vi "process.vi"(8 "error in (no error)":errorcluster, 11 "VI in":refnum<class "VI.lvclass">) -> (0 "error out":errorcluster, 3 "VI out":refnum<class "VI.lvclass">)   [LabVIEW 2016, in "VI.lvclass"]
uses:
  VI.lvclass
  C:/LSST_TS/SystemSW/ct_tools/ProjectItem/ProjectItem.lvclass
  ProjectItem/ProjectItem.lvclass/ProjectItem.ctl
  ProjectItem/ProjectItem.lvclass
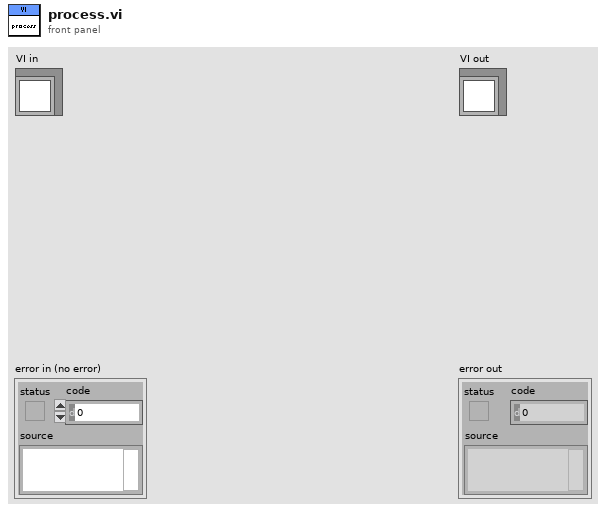
[diagram p1: front panel]
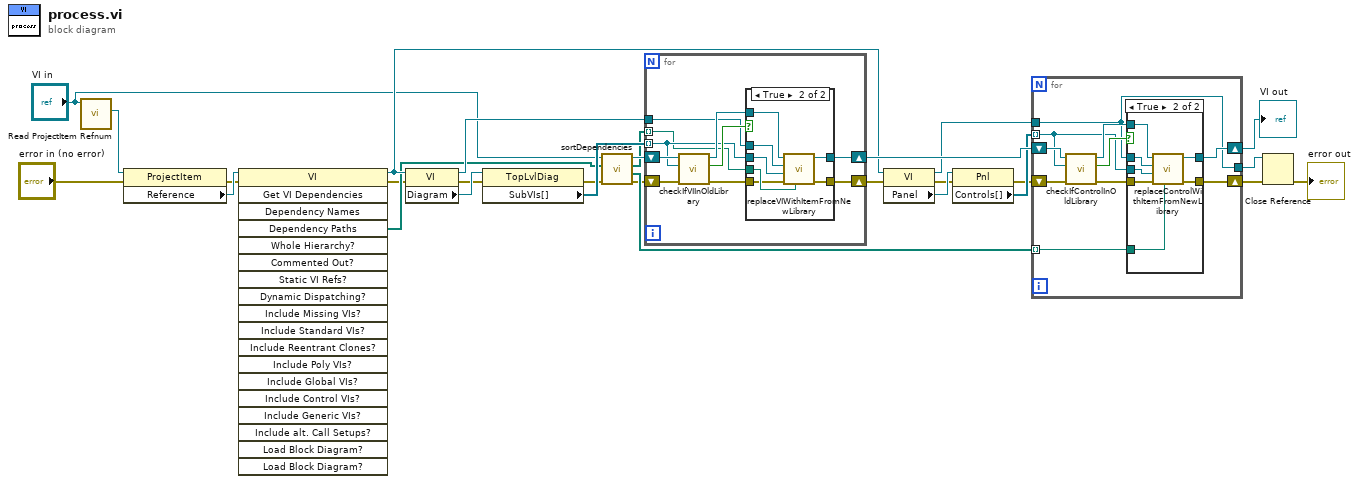
[diagram p0: block diagram]
diagram:
  n1 = call "Read ProjectItem Refnum.vi"("ProjectItem in"="VI in") -> ("ProjectItem Refnum"=w26:refnum<vi>)  [unwired: 9 in, 1 out]
  n2 = property class="ProjectItem"(reference=w26, error in="error in (no error)") -> (error out=w11:errorcluster, "Reference"=w25:refnum<vi>)  [unwired: 1 out]
  n3 = invoke class="VI" method="Get VI Dependencies"(reference=w25, error in=w11) -> (reference out=w20:refnum<vi>, error out=w10:errorcluster, "Dependency Paths"=w15:path[])  [unwired: 17 in, 16 out]
  n4 = property class="VI"(reference=w20, error in=w10) -> (reference out=w24:refnum<vi>, error out=w9:errorcluster, "Diagram"=w28:refnum<vi>)
  n5 = property class="TopLvlDiag"(reference=w28, error in=w9) -> (error out=w8:errorcluster, "SubVIs[]"=w27:refnum<vi>[])  [unwired: 1 out]
  n6 = call "sortDependencies.vi"("error in (no error)"=w8, "Dependency Paths"=w15, "VI in"="VI in") -> ("error out"=w7:errorcluster, "ControlDependencyPaths"=w13:path[], "VIDependencyPaths"=w14:path[], "VI out"=w16:refnum<class "VI.lvclass">)  [unwired: 5 in]
  n7 = for {
    shift-right: [w36] -> w22
    shift-left: w16 -> [w38]
    tunnel: w27 -> [w33] mode=indexing
    tunnel: w24 -> [w34]
    tunnel: w14 -> [w32] mode=indexing
    shift-right: [w29] -> w6
    shift-left: w7 -> [w31]
    n8 = call "checkIfVIInOldLibrary.vi"("error in (no error)"=w31, "element"=w33, "VI in"=w38) -> ("error out"=w30:errorcluster, "isMemberOfOldLibrary"=w35:bool, "VI out"=w37:refnum<class "VI.lvclass">)  [unwired: 5 in, 1 out]
    n9 = case shown="True" w35 {
      tunnel: w37 -> [w40 w47]
      tunnel: [w40 w46] -> w36
      tunnel: w34 -> [_ w45]
      tunnel: w33 -> [_ w44]
      tunnel: w32 -> [_ w43]
      tunnel: w30 -> [w39 w42]
      tunnel: [w39 w41] -> w29
      frame False {
      }
      frame True {
        n10 = call "replaceVIWithItemFromNewLibrary.vi"("SubVI Path"=w43, "error in (no error)"=w42, "SubVI Refnum"=w44, "Calling VI Reference"=w45, "VI in"=w47) -> ("error out"=w41:errorcluster, "VI out"=w46:refnum<class "VI.lvclass">)  [unwired: 5 in]
      }
    }
  }
  n11 = property class="VI"(reference=w20, error in=w6) -> (reference out=w19:refnum<vi>, error out=w5:errorcluster, "Panel"=w21:refnum<vi>)
  n12 = property class="Pnl"(reference=w21, error in=w5) -> (error out=w4:errorcluster, "Controls[]"=w18:refnum<vi>[])  [unwired: 1 out]
  n13 = for {
    shift-right: [w55] -> w23
    shift-left: w22 -> [w57]
    tunnel: w19 -> [w48]
    tunnel: w13 -> [w53] mode=indexing
    tunnel: w18 -> [w52] mode=indexing
    shift-right: [w49] -> w2
    shift-left: w4 -> [w51]
    tunnel: [w48] -> w3
    n14 = call "checkIfControlInOldLibrary.vi"("error in (no error)"=w51, "Ctl Refnum"=w52, "VI in"=w57) -> ("error out"=w50:errorcluster, "isMemberOfOldLibrary"=w54:bool, "VI out"=w56:refnum<class "VI.lvclass">)  [unwired: 5 in, 1 out]
    n15 = case shown="True" w54 {
      tunnel: w56 -> [w59 w66]
      tunnel: [w59 w65] -> w55
      tunnel: w48 -> [_ w60]
      tunnel: w52 -> [_ w64]
      tunnel: w53 -> [_ w63]
      tunnel: w50 -> [w58 w62]
      tunnel: [w58 w61] -> w49
      frame False {
      }
      frame True {
        n16 = call "replaceControlWithItemFromNewLibrary.vi"("SubVI Path"=w63, "error in (no error)"=w62, "Ctl Refnum"=w64, "Calling VI Reference"=w60, "VI in"=w66) -> ("error out"=w61:errorcluster, "VI out"=w65:refnum<class "VI.lvclass">)  [unwired: 5 in]
      }
    }
  }
  "VI out" <- w23
  n17 = Close Reference(reference=w3, error in (no error)=w2) -> (error out=→"error out":errorcluster)
